vi "Teleop.vi"(10 "Match Info":T1={"Autonomous Elapsed Seconds"=0.0, "TeleOp Elapsed Seconds"=0.0, "Disabled Elapsed Seconds"=0.0, "Visited Autonomous"=FALSE, "Visited TeleOp"=FALSE, "Visited Disabled"=FALSE, "Autonomous Settings"={"Autonomous Style"=enum."Independent", "VI Refnum"=refnum}}, 11 "Call Context":T2) -> ()   [LabVIEW 2017]
doc: "This VI is called for each TeleOp packet received from the DS where the robot is not disabled. It is often used to read from the joysticks and update I/O or to update setpoints for timed control loops. It should complete and return within 20 milliseconds or it may miss DS packets."
uses:
  <vilib>/Rock Robotics/WPI/DriverStation/WPI_DriverStationDerivedRobotMode.ctl
  <vilib>/Rock Robotics/WPI/DriverStation/WPI_DriverStationMatch Info.ctl
  PowerUpSrc/Global_Var-RefNum/Joystick_Control.vi
  ArgosLib/ArgosLib.lvlib
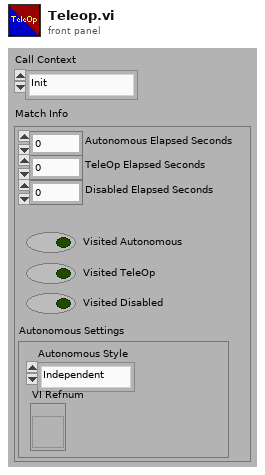
[diagram p1: front panel]
types:
  T1 = typedef "WPI_DriverStationMatch Info.ctl" = cluster{"Autonomous Elapsed Seconds":dbl, "TeleOp Elapsed Seconds":dbl, "Disabled Elapsed Seconds":dbl, "Visited Autonomous":bool, "Visited TeleOp":bool, "Visited Disabled":bool, "Autonomous Settings":cluster{"Autonomous Style":enum16{"Iterative", "Independent"}, "VI Refnum":refnum<vi>}}
  T2 = typedef "WPI_DriverStationDerivedRobotMode.ctl" = enum16{"Init", "Execute", "Stop"}
  T3 = typedef "RobotJoysticks.ctl" = cluster{"Driver Controller":T4, "Operator Controller":T4}
  T4 = typedef "WPI_JoystickDevRef.ctl" = cluster{"Device":T5}
  T5 = typedef "WPI_JoystickDeviceEnum.ctl" = enum16{"USB 0", "USB 1", "USB 2", "USB 3", "USB 4", "USB 5"}
  T6 = typedef "ArgosLib.lvlib/XBoxAxes_Type.ctl" = cluster{"Left_Trigger":dbl, "Right_Trigger ":dbl, "Left_X":dbl, "Left_Y":dbl, "Right_X":dbl, "Right_Y":dbl}
  T7 = typedef "ArgosLib.lvlib/XBoxButtons_Type.ctl" = cluster{"A":bool, "B":bool, "X":bool, " Y":bool, "LB":bool, " RB":bool, "Left_Thumb_Button":bool, "Right_Thumb_Button":bool, "Back":bool, "Start":bool, "Top":bool, "Right":bool, "Bottom":bool, "Left":bool}
  T8 = typedef "JoystickControls.ctl" = cluster{"drive speed":dbl, "drive turning":dbl, "Unassigned_LX":dbl, "Unassigned_RY":dbl, "Cube Release":bool, "Intake Forward":dbl, "Intake Reverse ":dbl, "Switch":bool, "Scale Low":bool, "Scale High":bool, "Shift":bool, "Arm To Preset":bool, "Unassigned_LJ":bool, "Unassigned_RJ":bool, "Swap_Back":bool, "Swap_Start":bool, "Arm Extend/Retract":dbl, "Unassigned_RX 2":dbl, "Unassigned_LX 2":dbl, "Arm  Pivot Up/Down ":dbl, "Cube Release 2":bool, "Extend/Retract Intake":dbl, "Open/Close Intake":dbl, "Switch 2":bool, "Scale High 2":bool, "Scale Low 2":bool, "Claw Pinch 2":bool, "Unassigned_RB 2":bool, "Unassigned_LJ 2":bool, "Unassigned_RJ 2":bool, "Swap_Back 2":bool, "Swap_Start 2":bool, "Climb Up 2":bool, "Unassigned_Right 2":bool, "Climb Down 2":bool, "Unassigned_Left 2":bool, "Climb Up ":bool, " Unassigned_Right":bool, "Climb Down":bool, "Unassigned_Left":bool}
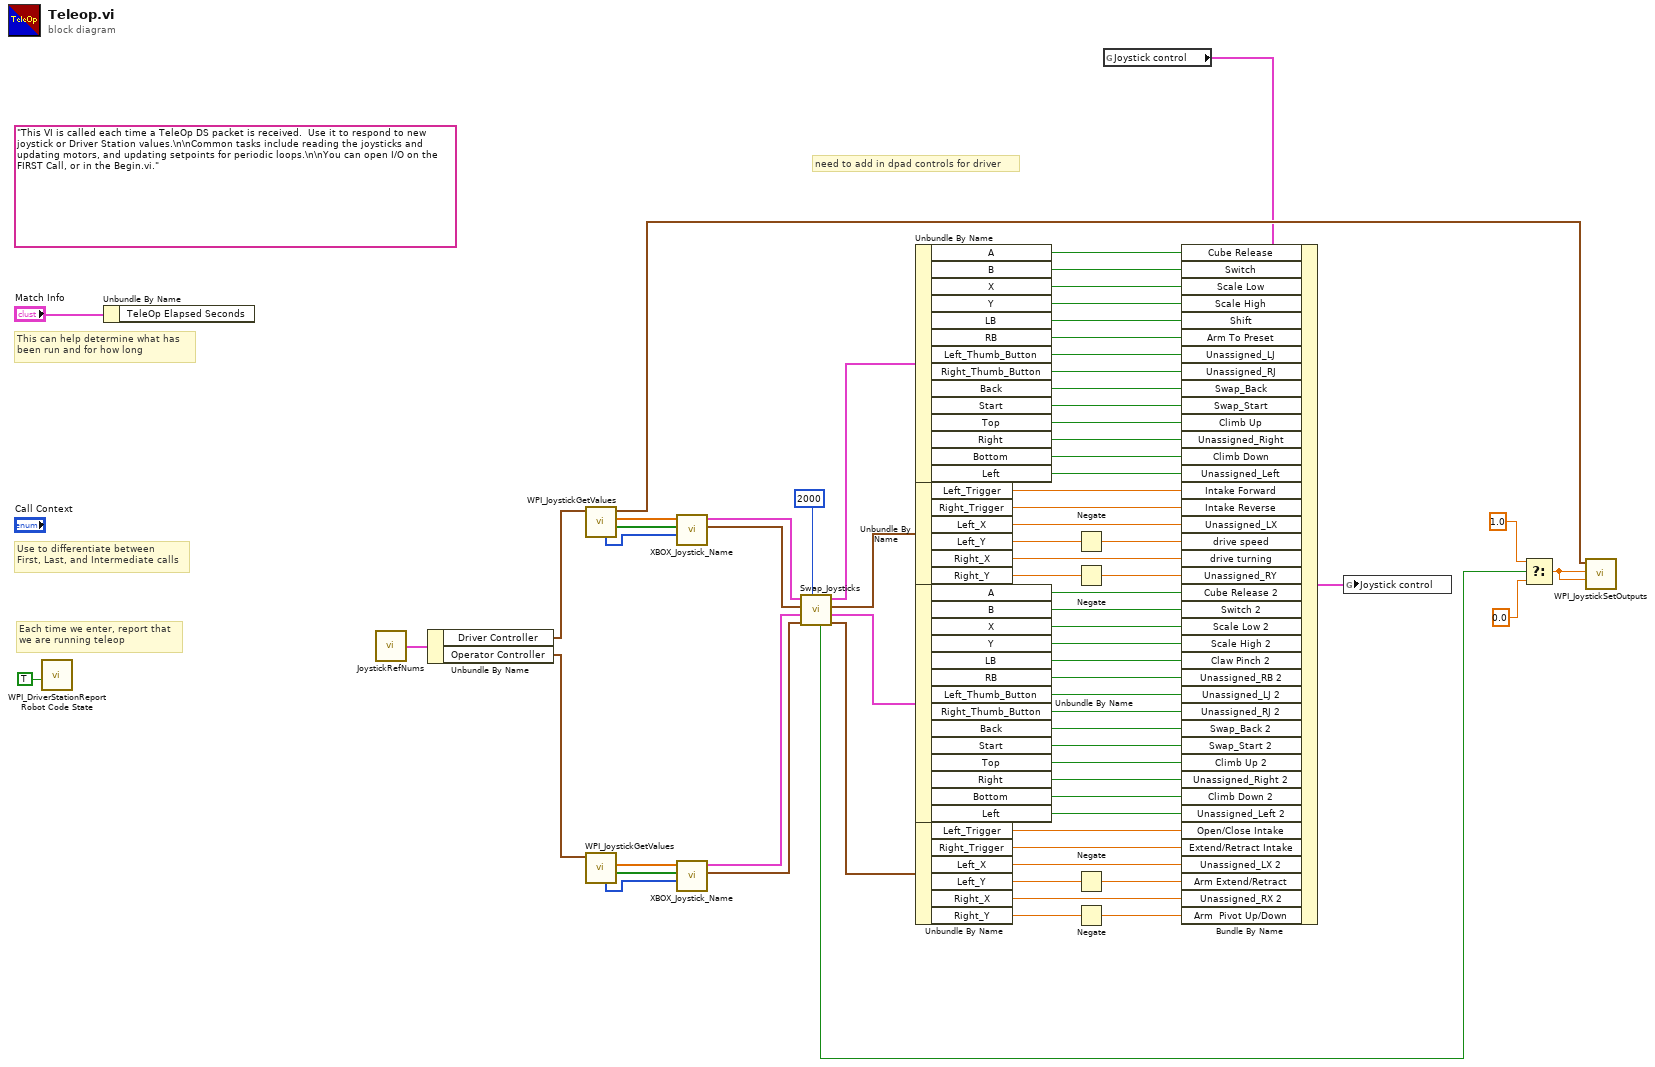
[diagram p0: block diagram]
diagram:
  (unwired) "This VI is called each time a TeleOp DS packet is received.  Use it to respond to new joystick or Driver Station values.\n\nCommon tasks include reading the joysticks and updating motors, and updating setpoints for periodic loops.\n\nYou can open I/O on the FIRST Call, or in the Begin.vi."
  # "need to add in dpad controls for driver"
  # "Each time we enter, report that\nwe are running teleop"
  # "Use to differentiate between\nFirst, Last, and Intermediate calls"
  # "This can help determine what has\nbeen run and for how long"
  n1 = call <vilib>:"WPI_DriverStationReport Robot Code State.vi"("TeleOp"=TRUE ("Autonomous")) -> ()  [unwired: 10 in, 1 out]
  n2 = Unbundle By Name("Match Info") -> ()  [unwired: 1 out]
  n3 = call "JoystickRefNums.vi"() -> ("Joysticks"=w50:T3)  [unwired: 1 in]
  n4 = Unbundle By Name(w50) -> ("Driver Controller"=w49:T4, "Operator Controller"=w48:T4)
  n5 = call <vilib>:"WPI_JoystickGetValues.vi"("JoystickDevRef"=w49) -> ("Buttons"=w68:bool[], "Axes"=w69:dbl[], "JoystickDevRef"=w59:T4, "POVs"=w47:i16[])  [unwired: 6 in, 1 out]
  n6 = call <vilib>:"WPI_JoystickGetValues.vi"("JoystickDevRef"=w48) -> ("Buttons"=w67:bool[], "Axes"=w66:dbl[], "POVs"=w46:i16[])  [unwired: 6 in, 2 out]
  n7 = call "XBOX_Joystick_Name.vi"("POVs"=w47, "Buttons"=w68, "Axes"=w69) -> ("Named Axes"=w55:T6, "Named Buttons"=w56:T7)  [unwired: 7 in]
  n8 = call "XBOX_Joystick_Name.vi"("POVs"=w46, "Buttons"=w67, "Axes"=w66) -> ("Named Axes"=w58:T6, "Named Buttons"=w57:T7)  [unwired: 7 in]
  n9 = call "Swap_Joysticks.vi"("Hold Time(ms)"=u32 2000, "Axes 1 In"=w58, "Buttons 1"=w57, "Axes 0 in"=w55, "Buttons 0"=w56) -> ("Axes 1 out"=w53:T6, "Buttons 1 out"=w52:T7, "Axes 0 out"=w51:T6, "Buttons 0 Out"=w54:T7, "Swap?"=w61:bool)
  n10 = Unbundle By Name(w54) -> ("A"=w44:bool, "B"=w43:bool, "X"=w42:bool, "Y"=w41:bool, "LB"=w40:bool, "RB"=w39:bool, "Left_Thumb_Button"=w38:bool, "Right_Thumb_Button"=w37:bool, "Back"=w36:bool, "Start"=w35:bool, "Top"=w34:bool, "Right"=w33:bool, "Bottom"=w32:bool, "Left"=w31:bool)
  n11 = Unbundle By Name(w51) -> ("Left_Trigger"=w30:dbl, "Right_Trigger"=w29:dbl, "Left_X"=w28:dbl, "Left_Y"=w27:dbl, "Right_X"=w25:dbl, "Right_Y"=w24:dbl)
  n12 = Unbundle By Name(w52) -> ("A"=w22:bool, "B"=w21:bool, "X"=w20:bool, "Y"=w19:bool, "LB"=w18:bool, "RB"=w17:bool, "Left_Thumb_Button"=w16:bool, "Right_Thumb_Button"=w15:bool, "Back"=w14:bool, "Start"=w13:bool, "Top"=w12:bool, "Right"=w11:bool, "Bottom"=w10:bool, "Left"=w9:bool)
  n13 = Unbundle By Name(w53) -> ("Left_Trigger"=w8:dbl, "Right_Trigger"=w7:dbl, "Left_X"=w6:dbl, "Left_Y"=w5:dbl, "Right_X"=w3:dbl, "Right_Y"=w4:dbl)
  n14 = Negate(x=w27) -> (-x=w26:dbl)
  n15 = Negate(x=w24) -> (-x=w23:dbl)
  n16 = Negate(x=w5) -> (-x=w2:dbl)
  n17 = Negate(x=w4) -> (-x=w1:dbl)
  n18 = global read "Joystick_Control.vi" "Joystick control"() -> (w45:T8)
  n19 = Bundle By Name(cluster=w45, "Cube Release"=w44, "Switch"=w43, "Scale Low"=w42, "Scale High"=w41, "Shift"=w40, "Arm To Preset"=w39, "Unassigned_LJ"=w38, "Unassigned_RJ"=w37, "Swap_Back"=w36, "Swap_Start"=w35, "Climb Up"=w34, "Unassigned_Right"=w33, "Climb Down"=w32, "Unassigned_Left"=w31, "Intake Forward"=w30, "Intake Reverse"=w29, "Unassigned_LX"=w28, "drive speed"=w26, "drive turning"=w25, "Unassigned_RY"=w23, "Cube Release 2"=w22, "Switch 2"=w21, "Scale Low 2"=w20, "Scale High 2"=w19, "Claw Pinch 2"=w18, "Unassigned_RB 2"=w17, "Unassigned_LJ 2"=w16, "Unassigned_RJ 2"=w15, "Swap_Back 2"=w14, "Swap_Start 2"=w13, "Climb Up 2"=w12, "Unassigned_Right 2"=w11, "Climb Down 2"=w10, "Unassigned_Left 2"=w9, "Open/Close Intake"=w8, "Extend/Retract Intake"=w7, "Unassigned_LX 2"=w6, "Arm Extend/Retract"=w2, "Unassigned_RX 2"=w3, "Arm  Pivot Up/Down"=w1) -> (w65:T8)
  n20 = global write "Joystick_Control.vi" "Joystick control"(w65) -> ()
  n21 = Select(t=1.0, s=w61, f=0.0) -> (s? t:f=w64:dbl)
  n22 = call <vilib>:"WPI_JoystickSetOutputs.vi"("Right Rumble"=w64, "Left Rumble"=w64, "JoystickDevRef"=w59) -> ()  [unwired: 7 in, 2 out]
